vi "Alignment.vi"(0 "Range":dbl format="%#_13g", 1 "Target":dbl format="%#_13g", 2 "Gyroscope Angle":dbl format="%#_13g", 3 "RightMotorSpeed":dbl format="%#_13g", 4 "LeftMotorSpeed":dbl format="%#_13g", 5 "POV":i32) -> (15 "Right Motor":dbl format="%#_13g", 17 "LeftAndRight?":bool, 18 "Left Motor":dbl format="%#_13g")   [LabVIEW 2016]
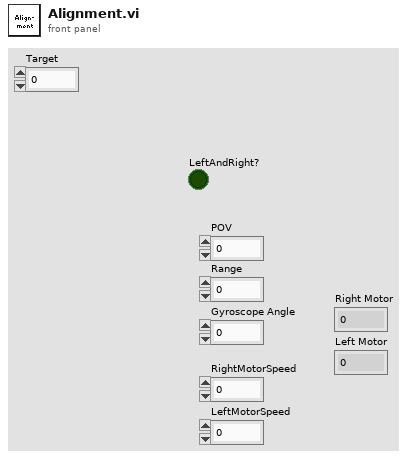
[diagram p1: front panel]
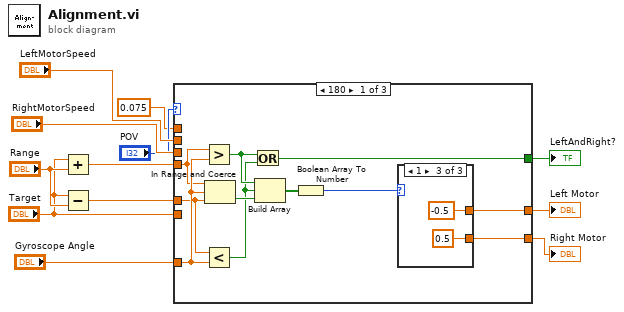
[diagram p0: block diagram]
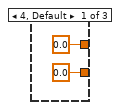
[diagram p2: hidden frame]
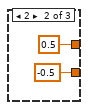
[diagram p3: hidden frame]
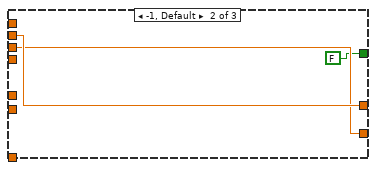
[diagram p4: hidden frame]
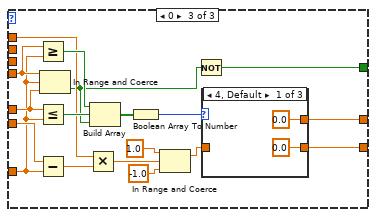
[diagram p5: hidden frame]
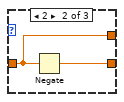
[diagram p6: hidden frame]
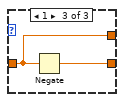
[diagram p7: hidden frame]
diagram:
  n1 = Add(x="Target", y="Range") -> (x+y=w6:dbl)
  n2 = Subtract(x="Target", y="Range") -> (x-y=w5:dbl)
  n3 = case shown="180" "POV" {
    tunnel: [w17 w32 w46] -> w12
    tunnel: "LeftMotorSpeed" -> [_ w32 _]
    tunnel: [w18 w31 w47] -> w10
    tunnel: "RightMotorSpeed" -> [_ w31 _]
    tunnel: "Gyroscope Angle" -> [w20 _ w41]
    tunnel: w6 -> [w16 _ w45]
    tunnel: w5 -> [w19 _ w50]
    tunnel: [w14 FALSE w33] -> w3
    tunnel: "Target" -> [_ _ w42]
    tunnel: 0.075 -> [_ _ w39]
    frame 180 {
      n4 = Greater?(x=w16, y=w20) -> (0:w15:bool)
      n5 = Less?(x=w19, y=w20) -> (x < y?=w13:bool)
      n6 = In Range and Coerce(upper limit=w16, x=w20, lower limit=w19) -> (In Range?=w23:bool)  [unwired: 1 out]
      n7 = Or(x=w15, y=w13) -> (x .or. y?=w14:bool)
      n8 = Build Array(w15, w13, w23) -> (w22:bool[])
      n9 = Boolean Array To Number(Boolean array=w22) -> (number=w21:u32)
      n10 = case shown="1" w21 {
        tunnel: [0.0 -0.5 0.5] -> w18
        tunnel: [0.0 0.5 -0.5] -> w17
        frame 4, Default {
        }
        frame 2 {
        }
        frame 1 {
        }
      }
    }
    frame -1, Default {
    }
    frame 0 {
      n11 = Greater Or Equal?(x=w45, y=w41) -> (x >= y?=w44:bool)
      n12 = Less Or Equal?(x=w50, y=w41) -> (x <= y?=w43:bool)
      n13 = Subtract(x=w42, y=w41) -> (x-y=w40:dbl)
      n14 = In Range and Coerce(upper limit=w45, x=w41, lower limit=w50) -> (In Range?=w34:bool)  [unwired: 1 out]
      n15 = Multiply(x=w39, y=w40) -> (x*y=w38:dbl)
      n16 = Build Array(w44, w43, w34) -> (w49:bool[])
      n17 = Boolean Array To Number(Boolean array=w49) -> (number=w48:u32)
      n18 = In Range and Coerce(upper limit=1.0, x=w38, lower limit=-1.0) -> (coerced(x)=w37:dbl)  [unwired: 1 out]
      n19 = Not(x=w34) -> (.not. x?=w33:bool)
      n20 = case shown="4, Default" w48 {
        tunnel: [0.0 w53 w55] -> w47
        tunnel: [0.0 w54 w56] -> w46
        tunnel: w37 -> [_ w54 w56]
        frame 4, Default {
        }
        frame 2 {
          n21 = Negate(x=w54) -> (-x=w53:dbl)
        }
        frame 1 {
          n22 = Negate(x=w56) -> (-x=w55:dbl)
        }
      }
    }
  }
  "Left Motor" <- w12
  "Right Motor" <- w10
  "LeftAndRight?" <- w3
